vi "Agilent 34970 Read Chans in Scan List.vi"(8 "error in (no error)":errorcluster, 11 "VISA Resource Name":refnum<visa-resource-name>) -> (0 "error out":errorcluster, 2 "Values Array":dbl[](array[numeric]) format="%.2f", 3 "VISA Resource Name Out":refnum<visa-resource-name>)   [LabVIEW 2016]
uses:
  Agilent 34970.lvlib
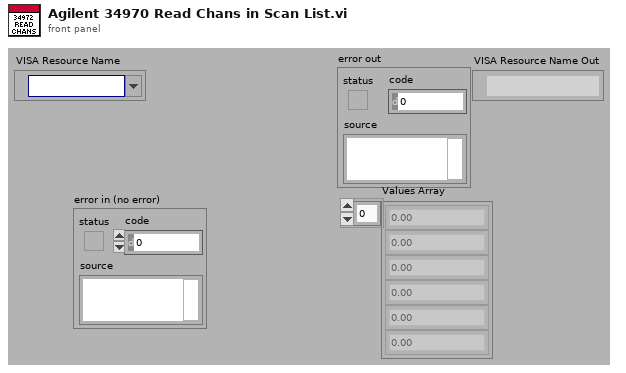
[diagram p1: front panel]
types:
  T1 = enum16{"Enable Register", "Event Register", "Operation Complete Bit"}
  T2 = enum16{"Manual", "Minimum", "Maximum", "Infinity"}
  T3 = enum16{"Bus", "Immediate", "External", "Alarm 1", "Alarm 2", "Alarm 3", "Alarm 4", "Timer"}
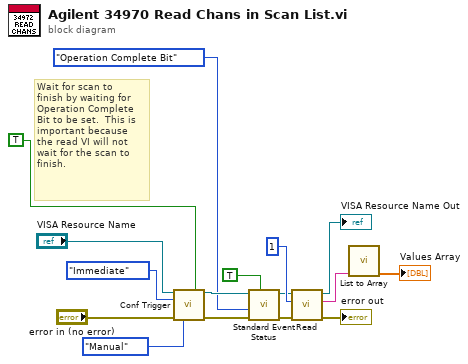
[diagram p0: block diagram]
diagram:
  # "Wait for scan to \nfinish by waiting for \nOperation Complete \nBit to be set.  This is\nimportant because\nthe read VI will not \nwait for the scan to\nfinish."
  n1 = call "Conf Trigger.vi"("VISA Resource Name"="VISA Resource Name", "Wait for Trigger? (F:No)"=TRUE, "Source (1:Immediate)"=T3."Immediate", "error in (no error)"="error in (no error)", "Max Trigger Count (3:Inf)"=T2."Manual") -> ("VISA Resource Name Out"=w15:refnum<visa-resource-name>, "error out"=w16:errorcluster)  [unwired: 8 in, 1 out]
  n2 = call "Standard Event Status.vi"("Set/Check? (F:Set)"=TRUE, "error in (no error)"=w16, "Check Parameter (0:Enable Reg)"=T1."Operation Complete Bit", "VISA Resource Name"=w15) -> ("error out"=w10:errorcluster, "VISA Resource Name Out"=w9:refnum<visa-resource-name>)  [unwired: 5 in, 1 out]
  n3 = call "Read.vi"("error in (no error)"=w10, "# Channels (1)"=1 ("# Channels (0)"), "VISA Resource Name"=w9) -> ("error out"=→"error out":errorcluster, "Readings"=w3:string, "VISA Resource Name Out"=→"VISA Resource Name Out":refnum<visa-resource-name>)  [unwired: 5 in, 1 out]
  n4 = call "List to Array.vi"("List (empty)"=w3) -> ("Output Number Array"=→"Values Array":dbl[])  [unwired: 9 in, 1 out]
